vi "CNTRLR - Fire Wash Entry.vi"(8 "error in (no error)":errorcluster, 10 "Wash Entry":bool, 11 "View Model":T1) -> (0 "error out":errorcluster)   [LabVIEW 2017]
doc: "Generates User Event = Wash Entry to Wash Display Console View."
uses:
  View Model/Controls/View Model.ctl
  View Model/Controls/Shared Model.ctl
  Error Handler/Controls/Error Model.ctl
  Error Handler/Controls/Error Message.ctl
  Error Handler/Controls/Error Level.ctl
  Configuration/Controls/Database Model.ctl
  Configuration/Controls/Database Message.ctl
  Configuration/Controls/Database Command.ctl
  Configuration/Controls/Database Overhead.ctl
  Configuration/Controls/Database Status.ctl
  Configuration/Controls/Database Record.ctl
  Controls/CNTRLR - Model.ctl
  Controls/CNTRLR - Message.ctl
  Controls/CNTRLR - Command.ctl
  Controls/CNTRLR - Overhead.ctl
  Controls/CNTRLR - Position.ctl
  Controls/CNTRLR - State.ctl
  Controls/CNTRLR - Wash Step.ctl
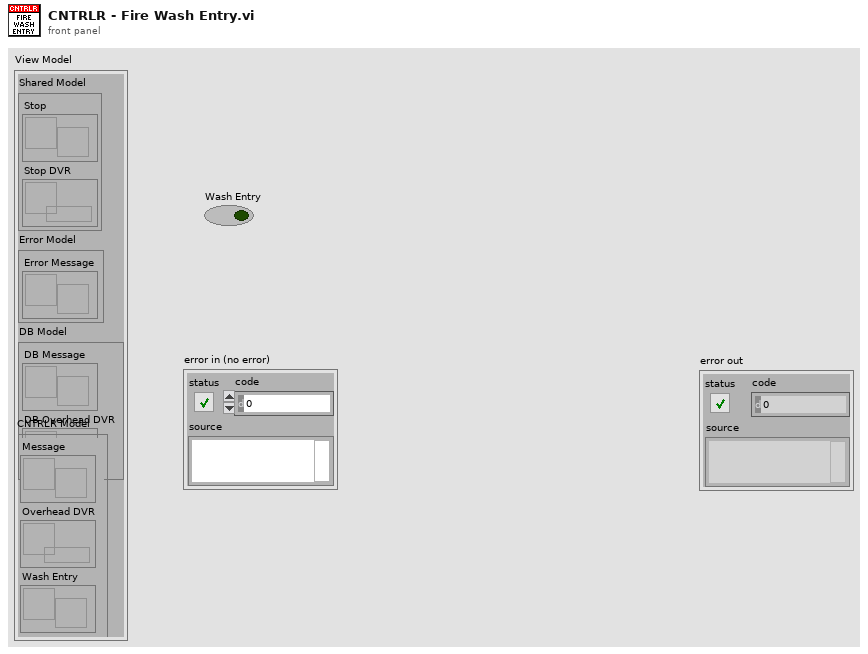
[diagram p1: front panel]
types:
  T1 = typedef "View Model.ctl" = cluster{"Shared Model":T2, "Error Model":T3, "DB Model":T4, "CNTRLR Model":T5}
  T2 = typedef "Shared Model.ctl" = cluster{"Stop":refnum<user-event>, "Stop DVR":refnum<data-value>}
  T3 = typedef "Error Model.ctl" = cluster{"Error Message":refnum<user-event>}
  T4 = typedef "Database Model.ctl" = cluster{"DB Message":refnum<user-event>, "DB Overhead DVR":refnum<data-value>}
  T5 = typedef "CNTRLR - Model.ctl" = cluster{"Message":refnum<user-event>, "Overhead DVR":refnum<data-value>, "Wash Entry":refnum<user-event>, "Out of Position":refnum<user-event>}
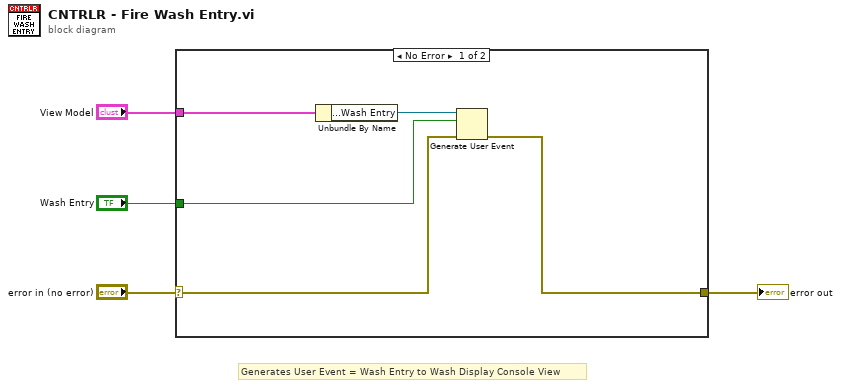
[diagram p0: block diagram]
diagram:
  # "Generates User Event = Wash Entry to Wash Display Console View"
  n1 = case shown="No Error" "error in (no error)" {
    selector: "error in (no error)" -> [w7 w10]
    tunnel: [w6 w10] -> w3
    tunnel: "View Model" -> [w9 _]
    tunnel: "Wash Entry" -> [w5 _]
    frame No Error {
      n2 = Unbundle By Name(w9) -> ("CNTRLR Model.Wash Entry"=w8:refnum<user-event>)
      n3 = Generate User Event(user event=w8, event data cluster=w5, error in=w7) -> (error out=w6:errorcluster)  [unwired: 1 in, 1 out]
    }
    frame Error {
    }
  }
  "error out" <- w3
